vi "Setting Powered ON Setup.vi"(8 "error in (no error)":errorcluster, 10 "Powered ON Setup (RST)":u16(ring) items=["RST", "SAV0", "SAV1", "SAV2", "SAV3", "SAV4"], 11 "VISA resource name":refnum<visa-resource-name>) -> (0 "error out":errorcluster, 3 "VISA resource name out":refnum<visa-resource-name>)   [LabVIEW 2020, in "Keithley 2450.lvlib"]
doc: "This selects the defaults that are used when instrument is powered on."
uses:
  <instrlib>/Keithley 2450/Keithley 2450.lvlib
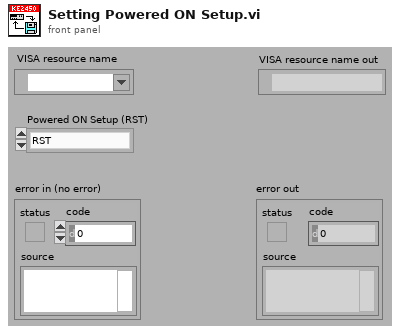
[diagram p1: front panel]
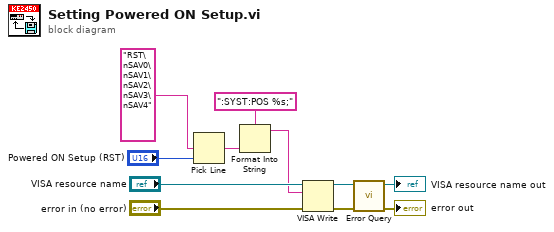
[diagram p0: block diagram]
diagram:
  n1 = Pick Line(multi-line string="RST\nSAV0\nSAV1\nSAV2\nSAV3\nSAV4", line index="Powered ON Setup (RST)") -> (output string=w3:string)  [unwired: 1 in]
  n2 = Format Into String(format string=":SYST:POS %s;", w3) -> (resulting string=w5:string)  [unwired: 2 in, 1 out]
  n3 = VISA Write(VISA resource name="VISA resource name", write buffer=w5, error in (no error)="error in (no error)") -> (VISA resource name out=w7:refnum<visa-resource-name>, error out=w6:errorcluster)  [unwired: 1 out]
  n4 = call <instrlib>:"Error Query.vi"("error in (no error)"=w6, "VISA resource name"=w7) -> ("error out"=→"error out":errorcluster, "VISA resource name out"=→"VISA resource name out":refnum<visa-resource-name>)  [unwired: 8 out]
